vi "pingTest.vi"(10 "IpAddress":string) -> (2 "Available":bool)   [LabVIEW 2014]
panel:
  out "standard output":string
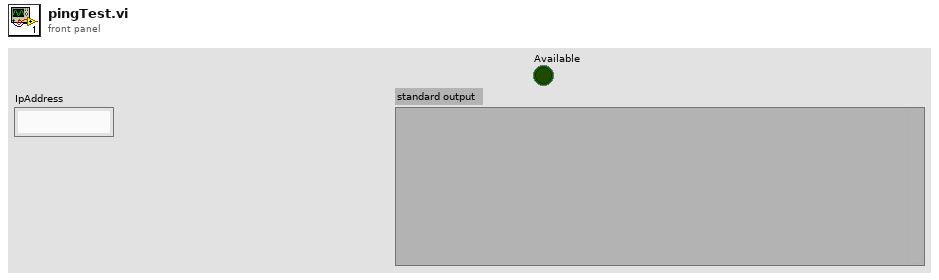
[diagram p1: front panel]
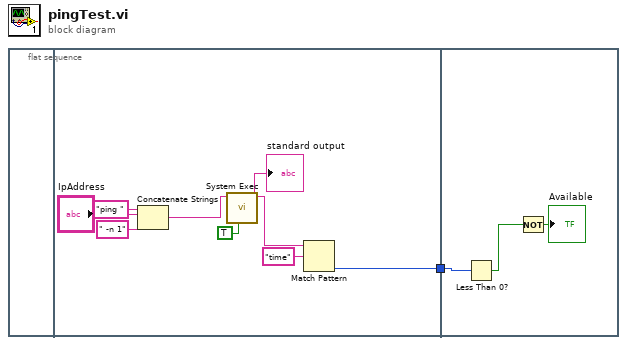
[diagram p0: block diagram]
diagram:
  n1 = flat-sequence {
    tunnel: [w2] -> w1
    tunnel: w1 -> [w11]
    frame #0 {
    }
    frame #1 {
      n2 = Concatenate Strings("ping " ("string"), "IpAddress", " -n 1" ("string")) -> (w5:string)
      n3 = call <vilib>:"System Exec.vi"("run minimized? (F)"=TRUE, "command line"=w5) -> ("standard output"=w4:string)  [unwired: 6 in, 3 out]
      "standard output" <- w4
      n4 = Match Pattern(string=w4, regular expression="time") -> (offset past match=w2:i32)  [unwired: 1 in, 3 out]
    }
    frame #2 {
      n5 = Less Than 0?(x=w11) -> (x < 0?=w10:bool)
      n6 = Not(x=w10) -> (.not. x?=→"Available":bool)
    }
  }
